vi "Periodic Tasks.vi"(8 "error in":errorcluster) -> ()   [LabVIEW 2017]
doc: "This VI runs in parallel to other robot code. It can contain as many user-defined periodic loops as you need. These can carry out PID or other sorts of timed response."
uses:
  <vilib>/Rock Robotics/WPI/Utilities/WPI_GetSetVariantRefNum.vi
  Robot Global Data.vi
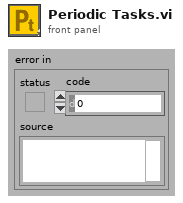
[diagram p1: front panel]
types:
  T1 = typedef "WPI_JoystickDevRef.ctl" = cluster{"Device":T2}
  T2 = typedef "WPI_JoystickDeviceEnum.ctl" = enum16{"USB 0", "USB 1", "USB 2", "USB 3", "USB 4", "USB 5"}
  T3 = typedef "WPI_SwitchDevRef.ctl" = cluster{"DevStatus":errorcluster, "DIO Channel":T4, "CntIndex":T5, "Normally Closed":bool}
  T4 = typedef "FPGA_DIOChannel.ctl" = enum8{"DIO 0", "DIO 1", "DIO 2", "DIO 3", "DIO 4", "DIO 5", "DIO 6", "DIO 7", "DIO 8", "DIO 9", "DIO MXP 0", "DIO MXP 1", "DIO MXP 2", "DIO MXP 3", "DIO MXP 4", "DIO MXP 5", "DIO MXP 6", "DIO MXP 7", "DIO MXP 8", "DIO MXP 9", "DIO MXP 10", "DIO MXP 11", "DIO MXP 12", "DIO MXP 13", "DIO MXP 14", "DIO MXP 15", "SPI Port CS1", "SPI Port CS2", "SPI Port CS3", "SPI Port MISO", "SPI Port MOSI", "Invalid"}
  T5 = typedef "FPGA_CounterCtrSystemIndex.ctl" = enum8{"Ctr 0", "Ctr 1", "Ctr 2", "Ctr 3", "Ctr 4", "Ctr 5", "Ctr 6", "Ctr 7", "Invalid"}
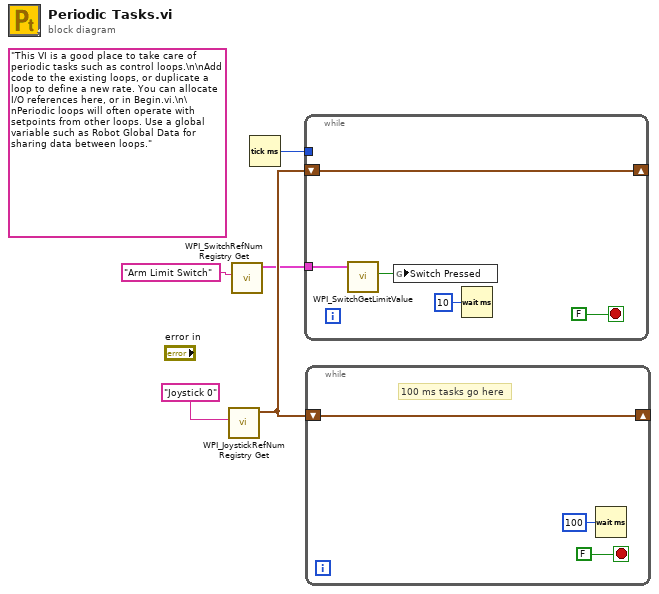
[diagram p0: block diagram]
diagram:
  (unwired) "This VI is a good place to take care of periodic tasks such as control loops.\n\nAdd code to the existing loops, or duplicate a loop to define a new rate. You can allocate I/O references here, or in Begin.vi.\n\nPeriodic loops will often operate with setpoints from other loops. Use a global variable such as Robot Global Data for sharing data between loops."
  n1 = call <vilib>:"WPI_JoystickRefNum Registry Get.vi"("refnum name"="Joystick 0") -> ("JoystickDevRef"=w4:T1)  [unwired: 1 in, 9 out]
  n2 = call <vilib>:"WPI_SwitchRefNum Registry Get.vi"("refnum name"="Arm Limit Switch") -> ("SwitchDevRef"=w1:T3)  [unwired: 9 in, 1 out]
  n3 = Tick Count (ms)() -> (millisecond timer value=w3:u32)
  n4 = while {
    shift-right: [w9] -> _
    shift-left: w4 -> [w9]
    tunnel: w3 -> [_]
    tunnel: w1 -> [w7]
    stop <- FALSE stop-if-true
    n5 = call <vilib>:"WPI_SwitchGetLimitValue.vi"("SwitchDevRef"=w7) -> ("Switch Pressed"=w6:bool)  [unwired: 8 in, 2 out]
    n6 = global write "Robot Global Data.vi" "Switch Pressed"(w6) -> ()
    n7 = Wait (ms)(milliseconds to wait=u32 10) -> ()  [unwired: 1 out]
  }
  n8 = while {
    shift-right: [w11] -> _
    shift-left: w4 -> [w11]
    stop <- FALSE stop-if-true
    # "100 ms tasks go here"
    n9 = Wait (ms)(milliseconds to wait=u32 100) -> ()  [unwired: 1 out]
  }
